vi "Get Min for Alarm.vi"(1 "Current Step Index":i32, 2 "Test Table":string[][](array[string]), 3 "Column Index for Min":i32=3) -> (0 "Min":dbl)   [LabVIEW 2018]
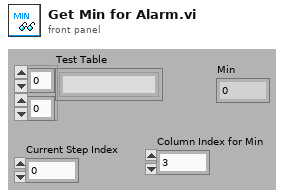
[diagram p1: front panel]
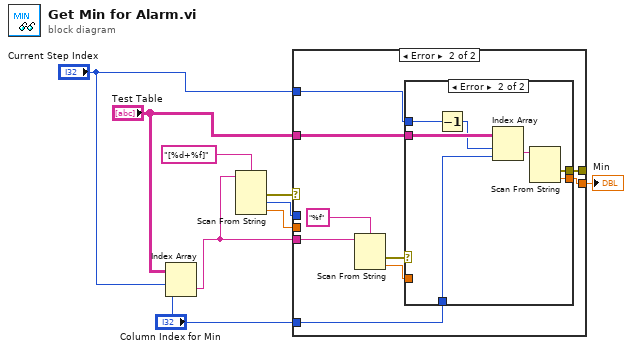
[diagram p0: block diagram]
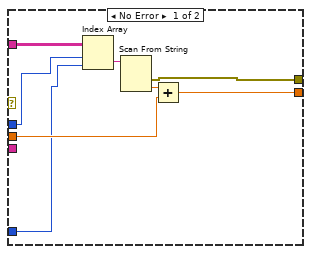
[diagram p2: hidden frame]
diagram:
  n1 = Index Array(array="Test Table", index (row)="Current Step Index", index (col)="Column Index for Min") -> (element=w2:string)
  n2 = Scan From String(format string="[%d+%f]", input string=w2) -> (error out=w5:errorcluster, output 1=w8:i32, output 2=w7:dbl)  [unwired: 4 in, 2 out]
  n3 = case shown="Error" w5 {
    tunnel: "Test Table" -> [w17 w23]
    tunnel: "Current Step Index" -> [_ w22]
    tunnel: w2 -> [_ w25]
    tunnel: w7 -> [w12 _]
    tunnel: [w13 w21] -> w9
    tunnel: w8 -> [w16 _]
    tunnel: "Column Index for Min" -> [w11 w19]
    tunnel: [w10 w18] -> _
    frame No Error {
      n4 = Index Array(array=w17, index (row)=w16, index (col)=w11) -> (element=w15:string)
      n5 = Scan From String(input string=w15) -> (error out=w10:errorcluster, output 1=w14:dbl)  [unwired: 4 in, 2 out]
      n6 = Add(x=w14, y=w12) -> (x+y=w13:dbl)
    }
    frame Error {
      n7 = Scan From String(format string="%f", input string=w25) -> (error out=w24:errorcluster, output 1=w20:dbl)  [unwired: 3 in, 2 out]
      n8 = case shown="Error" w24 {
        selector: w24 -> [w27 _]
        tunnel: w23 -> [_ w35]
        tunnel: w22 -> [_ w34]
        tunnel: [w28 w31] -> w21
        tunnel: w20 -> [w28 _]
        tunnel: w19 -> [_ w30]
        tunnel: [w27 w29] -> w18
        frame No Error {
        }
        frame Error {
          n9 = Decrement(x=w34) -> (x-1=w33:i32)
          n10 = Index Array(array=w35, index (row)=w33, index (col)=w30) -> (element=w32:string)
          n11 = Scan From String(input string=w32) -> (error out=w29:errorcluster, output 1=w31:dbl)  [unwired: 4 in, 2 out]
        }
      }
    }
  }
  "Min" <- w9
